vi "Copy (Data).vi"(7 "table \"path\"":string, 8 "error in (no error)":errorcluster, 9 "data":dbl[][](array[numeric]), 10 "column \"path\"(s) (empty=ALL)":string, 11 "Data.PGSQL":refnum<class "LV-Data.PGSQL.lvclass">) -> (0 "error out":errorcluster, 3 "Data.PGSQL out":refnum<class "LV-Data.PGSQL.lvclass">)   [LabVIEW 2019, in "LV-Data.PGSQL.lvclass"]
uses:
  LV-Data.PGSQL.lvclass
  <vilib>/JDP Science/PostgreSQL Library/Connection/PQ Connection.lvclass
  LV-Data.PGSQL.lvclass/LV-Data.PGSQL.ctl
panel:
  # "llab"
  # "time, column_path"
  # "new table"
  # "timestamps, data"
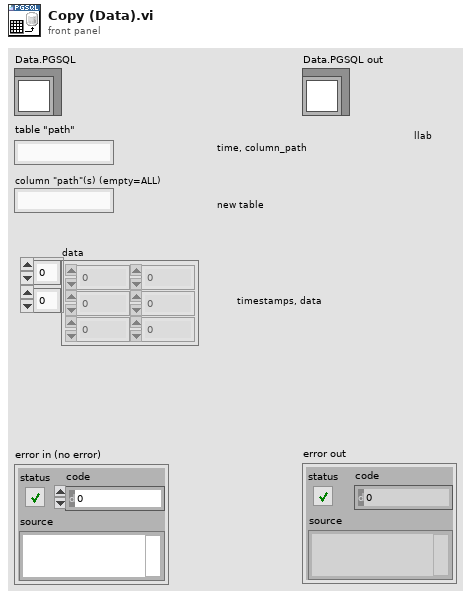
[diagram p1: front panel]
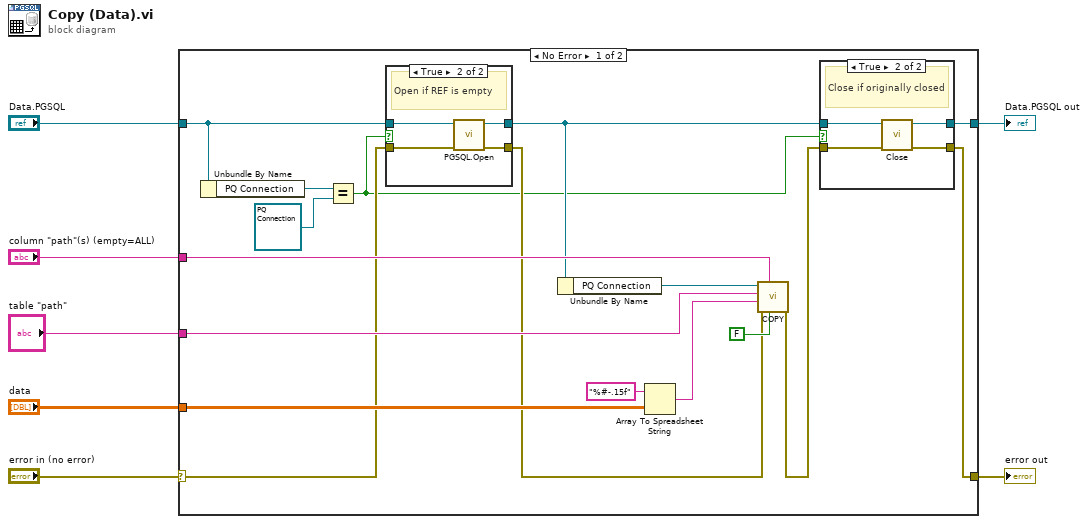
[diagram p0: block diagram]
diagram:
  n1 = case shown="No Error" "error in (no error)" {
    selector: "error in (no error)" -> [w10 w38]
    tunnel: "table \"path\"" -> [w22 _]
    tunnel: "Data.PGSQL" -> [w12 w37]
    tunnel: [w15 w38] -> w5
    tunnel: [w17 w37] -> w3
    tunnel: "data" -> [w19 _]
    tunnel: "column \"path\"(s) (empty=ALL)" -> [w18 _]
    frame No Error {
      n2 = Unbundle By Name(w12) -> ("PQ Connection"=w13:refnum<class "PQ Connection.lvclass">)
      n3 = Equal?(x=w13, y=refnum<class "PQ Connection.lvclass"> refnum ("PQ Connection")) -> (x = y?=w8:bool)
      n4 = case shown="True" w8 {
        tunnel: w12 -> [w25 w27]
        tunnel: [w25 w30] -> w11
        tunnel: [w26 w29] -> w9
        tunnel: w10 -> [w26 w28]
        frame False {
        }
        frame True {
          # "Open if REF is empty"
          n5 = call "PGSQL.Open.vi"("error in (no error)"=w28, "Data.PG in"=w27) -> ("error out"=w29:errorcluster, "Data.PG out"=w30:refnum<class "LV-Data.PGSQL.lvclass">)  [unwired: 8 in]
        }
      }
      n6 = Unbundle By Name(w11) -> ("PQ Connection"=w23:refnum<class "PQ Connection.lvclass">)
      n7 = Array To Spreadsheet String(array=w19, 3:"%#-.15f" ("format string")) -> (spreadsheet string=w20:string)  [unwired: 1 in]
      n8 = call <vilib>:"COPY.vi"("CSV?"=FALSE, "column name(s) (empty=ALL)"=w18, "error in (no error)"=w9, "buffer"=w20, "table name"=w22, "PQ Connection in"=w23) -> ("error out"=w16:errorcluster)  [unwired: 4 in, 1 out]
      n9 = case shown="True" w8 {
        tunnel: w11 -> [w31 w36]
        tunnel: w16 -> [w32 w35]
        tunnel: [w32 w34] -> w15
        tunnel: [w31 w33] -> w17
        frame False {
          # "Do not close if closed wasn't before"
        }
        frame True {
          # "Close if originally closed"
          n10 = call-dynamic "Close.vi"("error in (no error)"=w35, "Data.PG in"=w36) -> ("error out"=w34:errorcluster, "Data.PG out"=w33:refnum<class "LV-Data.PGSQL.lvclass">)  [unwired: 8 in]
        }
      }
    }
    frame Error {
    }
  }
  "error out" <- w5
  "Data.PGSQL out" <- w3
